vi "wheel_openclose.vi"(8 "error in (no error)":errorcluster, 10 "action":enum16{"open", "close"}(ring), 11 "thorlabs_FW102C in":refnum<class "thorlabs_FW102C.lvclass">) -> (0 "error out":errorcluster, 3 "thorlabs_FW102C out":refnum<class "thorlabs_FW102C.lvclass">)   [LabVIEW 2015, in "thorlabs_FW102C.lvclass"]
uses:
  thorlabs_FW102C.lvclass
  thorlabs_FW102C.lvclass/thorlabs_FW102C.ctl
  Thorlabs_FW102C.lvlib
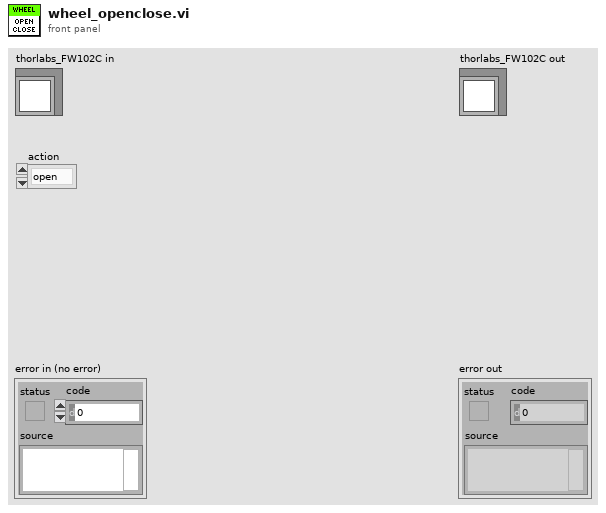
[diagram p1: front panel]
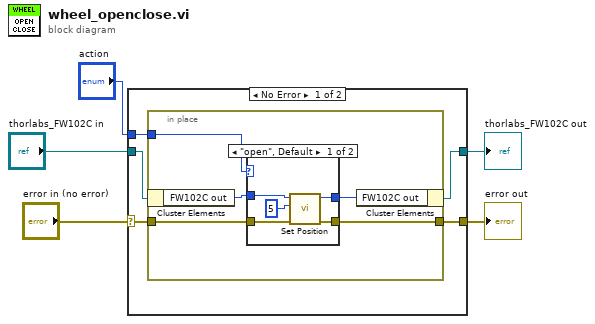
[diagram p0: block diagram]
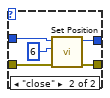
[diagram p2: hidden frame]
diagram:
  n1 = case shown="No Error" "error in (no error)" {
    selector: "error in (no error)" -> [w9 w27]
    tunnel: [w8 w27] -> w4
    tunnel: [w6 w26] -> w2
    tunnel: "thorlabs_FW102C in" -> [w10 w26]
    tunnel: "action" -> [w7 _]
    frame No Error {
      n2 = in-place {
        in-place-border: w9 -> [w13]
        in-place-border: [w12] -> w8
        in-place-border: w7 -> [w11]
        n3 = in-place-cluster #1(w10) -> ("FW102C out"=w15:i32)
        n4 = case shown="\"open\", Default" w11 {
          tunnel: w15 -> [w17 w25]
          tunnel: [w18 w24] -> w14
          tunnel: w13 -> [w20 w23]
          tunnel: [w19 w22] -> w12
          frame "open", Default {
            n5 = call "Set Position.vi"("error in (no error)"=w20, "Position"=5, "FW102C in"=w17) -> ("error out"=w19:errorcluster, "FW102C out"=w18:i32)  [unwired: 7 in]
          }
          frame "close" {
            n6 = call "Set Position.vi"("error in (no error)"=w23, "Position"=6, "FW102C in"=w25) -> ("error out"=w22:errorcluster, "FW102C out"=w24:i32)  [unwired: 7 in]
          }
        }
        n7 = in-place-cluster #1("FW102C out"=w14) -> (w6:refnum<class "thorlabs_FW102C.lvclass">)
      }
    }
    frame Error {
    }
  }
  "error out" <- w4
  "thorlabs_FW102C out" <- w2
